vi "probe_js.vi"() -> ()   [LabVIEW 2011]
uses:
  <vilib>/Utility/inputDevices.llb/joystickAcquire.vi
panel:
  out "axis info":T1
  out "nearest integer value":u8
  out "button info":T2
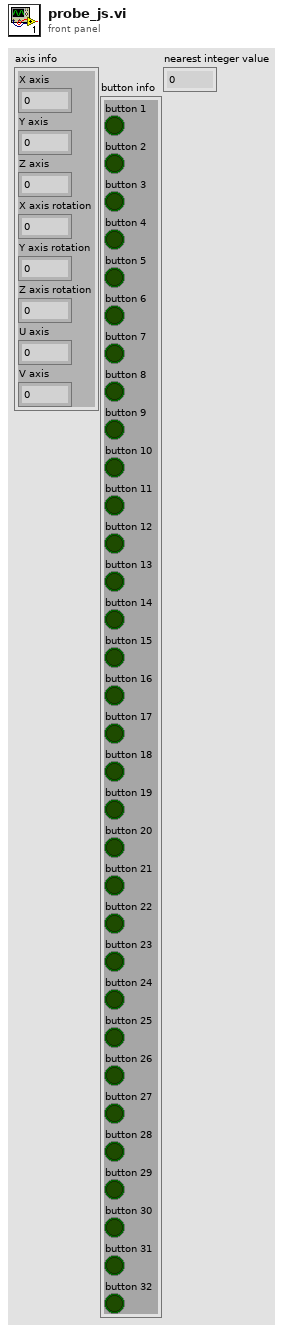
[diagram p1: front panel]
types:
  T1 = cluster{"X axis":dbl, "Y axis":dbl, "Z axis":dbl, "X axis rotation":dbl, "Y axis rotation":dbl, "Z axis rotation":dbl, "U axis":dbl, "V axis":dbl}
  T2 = cluster{"button 1":bool, "button 2":bool, "button 3":bool, "button 4":bool, "button 5":bool, "button 6":bool, "button 7":bool, "button 8":bool, "button 9":bool, "button 10":bool, "button 11":bool, "button 12":bool, "button 13":bool, "button 14":bool, "button 15":bool, "button 16":bool, "button 17":bool, "button 18":bool, "button 19":bool, "button 20":bool, "button 21":bool, "button 22":bool, "button 23":bool, "button 24":bool, "button 25":bool, "button 26":bool, "button 27":bool, "button 28":bool, "button 29":bool, "button 30":bool, "button 31":bool, "button 32":bool}
  T3 = cluster{"X axis":i32, "Y axis":i32, "Z axis":i32, "X axis rotation":i32, "Y axis rotation":i32, "Z axis rotation":i32, "U axis":i32, "V axis":i32}
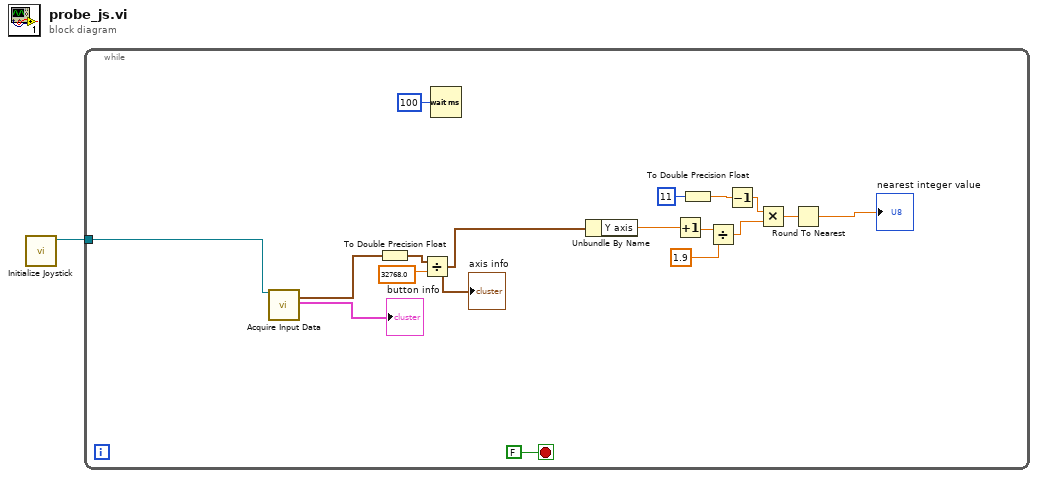
[diagram p0: block diagram]
diagram:
  n1 = call <vilib>:"Initialize Joystick.vi"() -> ("device ID"=w1:refnum<k1>)  [unwired: 10 in, 1 out]
  n2 = while {
    tunnel: w1 -> [w18]
    stop <- FALSE stop-if-true
    n3 = call-poly <vilib>:"Acquire Input Data.vi"("device ID"=w18) -> ("axis info"=w3:T3, "button info"=→"button info":T2)  [unwired: 14 in, 3 out]
    n4 = To Double Precision Float(number=w3) -> (double precision float=w4:T1)
    n5 = Divide(x=w4, y=32768.0) -> (x/y=w12:T1)
    "axis info" <- w12
    n6 = Wait (ms)(milliseconds to wait=u32 100) -> ()  [unwired: 1 out]
    n7 = Unbundle By Name(w12) -> ("Y axis"=w11:dbl)
    n8 = Increment(x=w11) -> (x+1=w10:dbl)
    n9 = To Double Precision Float(number=11) -> (double precision float=w14:dbl)
    n10 = Divide(x=w10, y=1.9) -> (x/y=w6:dbl)
    n11 = Decrement(x=w14) -> (x-1=w7:dbl)
    n12 = Multiply(x=w7, y=w6) -> (x*y=w8:dbl)
    n13 = Round To Nearest(number=w8) -> (nearest integer value=→"nearest integer value":dbl)
  }
